vi "Teleop Drivetrain Control.vi"(10 "Button Cluster":T1, 11 "Axes":T2) -> ()   [LabVIEW 2015]
uses:
  Common Code/Gamepads/Axes Cluster.ctl
  Common Code/Gamepads/Button Cluster.ctl
  Common Code/Change Detect.vi
  Common Code/Change Detect Boolean.vi
  Robot Global Data.vi
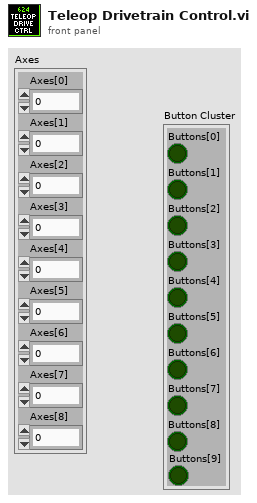
[diagram p1: front panel]
types:
  T1 = typedef "Button Cluster.ctl" = cluster{"Buttons[0]":bool, "Buttons[1]":bool, "Buttons[2]":bool, "Buttons[3]":bool, "Buttons[4]":bool, "Buttons[5]":bool, "Buttons[6]":bool, "Buttons[7]":bool, "Buttons[8]":bool, "Buttons[9]":bool}
  T2 = typedef "Axes Cluster.ctl" = cluster{"Axes[0]":dbl, "Axes[1]":dbl, "Axes[2]":dbl, "Axes[3]":dbl, "Axes[4]":dbl, "Axes[5]":dbl, "Axes[6]":dbl, "Axes[7]":dbl, "Axes[8]":dbl}
  T3 = typedef "Drivetrain Commands.ctl" = cluster{"Y Power":dbl, "Turn Power":dbl, "Distance":dbl, "1st Gear?":bool, "Modes":T4}
  T4 = typedef "Drivetrain Modes.ctl" = enum16{"Climb", "Manual", "Vision Targeting", "PID Distance Drive", "Hybrid"}
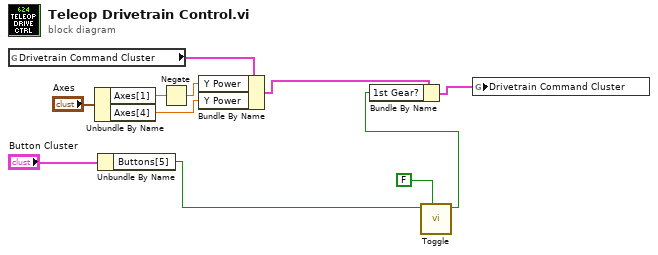
[diagram p0: block diagram]
diagram:
  n1 = global read "Robot Global Data.vi" "Drivetrain Command Cluster"() -> (w6:T3)
  n2 = Unbundle By Name("Axes") -> ("Axes[1]"=w9:dbl, "Axes[4]"=w7:dbl)
  n3 = Unbundle By Name("Button Cluster") -> ("Buttons[5]"=w5:bool)
  n4 = Negate(x=w9) -> (-x=w8:dbl)
  n5 = Bundle By Name(cluster=w6, "Y Power"=w8, "Y Power"=w7) -> (w3:T3)
  n6 = call "Toggle.vi"("Initial Value"=FALSE, "In"=w5) -> ("Toggled"=w2:bool)  [unwired: 9 in]
  n7 = Bundle By Name(cluster=w3, "1st Gear?"=w2) -> (w1:T3)
  n8 = global write "Robot Global Data.vi" "Drivetrain Command Cluster"(w1) -> ()
